vi "Gregorian day to Julian day Number.vi"(10 "Date (mm/dd/yyyy)":timestamp format="%<%X\n%x>T") -> (2 "output variable":dbl format="%#.0f")   [LabVIEW 2010]
uses:
  <vilib>/express/express arith-compare/Formula/XNode/ExpressFormulaBlockNode.xnode
panel:
  # "Select date and run program to get julianday number.\n\nIf you want to convert julianday number to normal date \nuse julian day number to  Grogorian date vi."
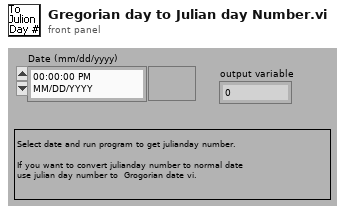
[diagram p1: front panel]
types:
  T1 = cluster{"second":i32, "minute":i32, "hour":i32, "day of month":i32, "month":i32, "year":i32, "day of week":i32, "day of year":i32, "is DST":i32}
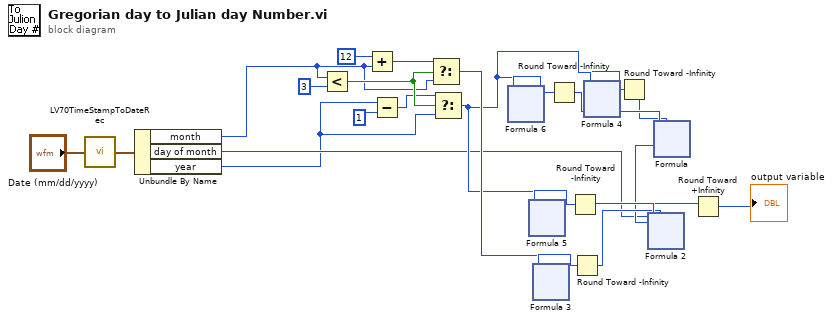
[diagram p0: block diagram]
diagram:
  n1 = call <vilib>:"LV70TimeStampToDateRec.vi"("time stamp"="Date (mm/dd/yyyy)") -> ("date time rec"=w4:T1)
  n2 = Unbundle By Name(w4) -> ("month"=w2:i32, "day of month"=w3:i32, "year"=w1:i32)
  n3 = Less?(x=w2, y=3) -> (x < y?=w21:bool)
  n4 = Add(x=12, y=w2) -> (x+y=w20:i32)
  n5 = Subtract(x=w1, y=1) -> (x-y=w19:i32)
  n6 = Select(t=w20, s=w21, f=w2) -> (s? t:f=w13:i32)
  n7 = Select(t=w19, s=w21, f=w1) -> (s? t:f=w12:i32)
  n8 = xnode "Formula 6"("j"=w12) -> ("Result"=w18:i32)  [unwired: 1 in, 1 out]
  n9 = xnode "Formula 5"("j"=w12) -> ("Result"=w17:i32)  [unwired: 1 in, 1 out]
  n10 = xnode "Formula 3"("m"=w13) -> ("Result"=w16:i32)  [unwired: 1 in, 1 out]
  n11 = Round Toward -Infinity(1:w18) -> (0:w10:i32)
  n12 = Round Toward -Infinity(1:w17) -> (0:w15:i32)
  n13 = Round Toward -Infinity(1:w16) -> (0:w14:i32)
  n14 = xnode "Formula 4"("j"=w12) -> ("Result"=w11:i32)  [unwired: 1 in, 1 out]
  n15 = Round Toward -Infinity(1:w11) -> (0:w9:i32)
  n16 = xnode "Formula"("x1"=w10, "x2"=w9) -> ("Result"=w8:i32)  [unwired: 1 in, 1 out]
  n17 = xnode "Formula 2"("j"=w15, "m"=w14, "d"=w3, "c"=w8) -> ("Result"=w7:i32)  [unwired: 1 in, 1 out]
  n18 = Round Toward +Infinity(x=w7) -> (ceil(x): smallest int >= x=→"output variable":i32)
